vi "Galil Motion Controller (Keith Koch's conflicted copy 2013-05-10).vi"   [LabVIEW 2011]
uses:
  _GlobalVariables&Libraries/ATV Program Global Variables.vi
types:
  T1 = cluster{"Drive Value Output String":string, "Steer Value Output String":string, "Error Out":errorcluster, "Initial Encoder Counts":string, "Disable Galil Terminal":bool, "Command Input":string}
  T2 = cluster{"End ATV Program":bool, "E-Stop":bool, "Save Logfile":bool, "Logfile Iteration Delay (ms)":u32, "Loop iteration time (ms)":u32, "Logfile Location":path, "Default GPS Navigation Path":path, "Computer":string, "Default GPS Boundary Path":path}
  T3 = cluster{"Navigation Coordinates":cluster{"Latitude":dbl, "Longitude":dbl}[], "Coordinate Count":u32, "Drive Speed":string, "Steer Angle":dbl, "Steering":dbl, "Direction to next Coordinate":dbl, "Drive":dbl, "Navigation Path":string}
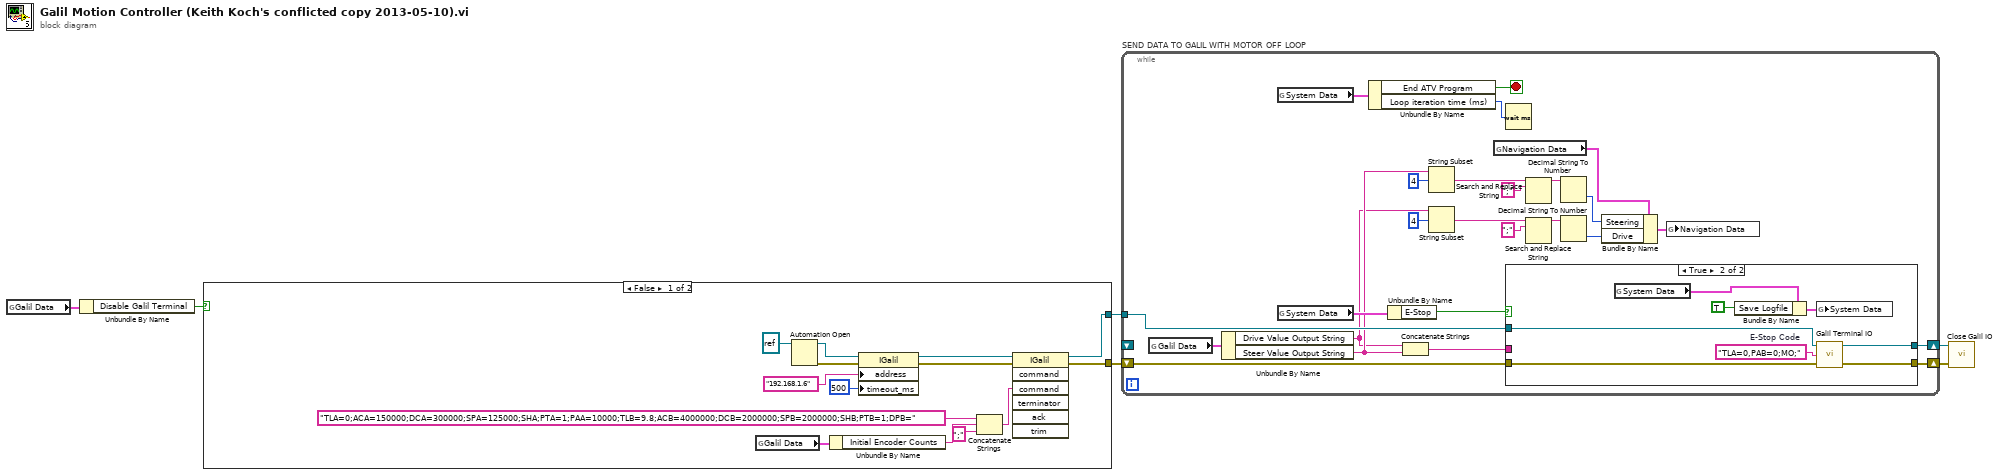
[diagram p0: block diagram]
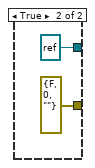
[diagram p2: hidden frame]
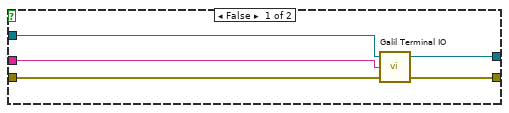
[diagram p3: hidden frame]
diagram:
  n1 = global read "ATV Program Global Variables.vi" "Galil Data"() -> (w4:T1)
  n2 = Unbundle By Name(w4) -> ("Disable Galil Terminal"=w3:bool)
  n3 = case shown="False" w3 {
    tunnel: [w14 refnum<k7> refnum ("Galil.IGalil")] -> w2
    tunnel: [w13 errorcluster {"status"=FALSE, "code"=0, "source"=""} ("error out")] -> w1
    frame False {
      n4 = global read "ATV Program Global Variables.vi" "Galil Data"() -> (w11:T1)
      n5 = Automation Open(Automation Refnum=refnum<k7> refnum ("Galil.IGalil")) -> (Automation Refnum=w19:refnum<k7>, error out=w18:errorcluster)  [unwired: 3 in]
      n6 = Unbundle By Name(w11) -> ("Initial Encoder Counts"=w10:string)
      n7 = property class="IGalil"(reference=w19, error in=w18, "address"="192.168.1.6", "timeout_ms"=500) -> (reference out=w8:refnum<k7>, error out=w7:errorcluster)
      n8 = Concatenate Strings("TLA=0;ACA=150000;DCA=300000;SPA=125000;SHA;PTA=1;PAA=10000;TLB=9.8;ACB=4000000;DCB=2000000;SPB=2000000;SHB;PTB=1;DPB=" ("Command Input"), w10, ";" ("string")) -> (w12:string)
      n9 = invoke class="IGalil" method="command"(reference=w8, error in=w7, "command"=w12) -> (reference out=w14:refnum<k7>, error out=w13:errorcluster)  [unwired: 4 in, 5 out]
    }
    frame True {
    }
  }
  n10 = while "SEND DATA TO GALIL WITH MOTOR OFF LOOP" {
    tunnel: w2 -> [w46]
    shift-right: [w43] -> w5
    shift-left: w1 -> [w44]
    shift-right: [w45] -> w6
    shift-left: _ -> [_]
    stop <- w38 stop-if-true
    n11 = global read "ATV Program Global Variables.vi" "Galil Data"() -> (w42:T1)
    n12 = Unbundle By Name(w42) -> ("Drive Value Output String"=w23:string, "Steer Value Output String"=w29:string)
    n13 = global read "ATV Program Global Variables.vi" "System Data"() -> (w39:T2)
    n14 = global read "ATV Program Global Variables.vi" "System Data"() -> (w41:T2)
    n15 = Unbundle By Name(w39) -> ("End ATV Program"=w38:bool, "Loop iteration time (ms)"=w37:u32)
    n16 = Unbundle By Name(w41) -> ("E-Stop"=w40:bool)
    n17 = Concatenate Strings(w23, w29) -> (w47:string)
    n18 = String Subset(string=w29, offset (0)=4) -> (substring=w34:string)  [unwired: 1 in]
    n19 = String Subset(string=w23, offset (0)=4) -> (substring=w27:string)  [unwired: 1 in]
    n20 = global read "ATV Program Global Variables.vi" "Navigation Data"() -> (w32:T3)
    n21 = Wait (ms)(milliseconds to wait=w37) -> ()  [unwired: 1 out]
    n22 = case shown="True" w40 {
      tunnel: w47 -> [w52 _]
      tunnel: w46 -> [w51 w58]
      tunnel: [w50 w60] -> w45
      tunnel: w44 -> [w49 w57]
      tunnel: [w48 w59] -> w43
      frame False {
        n23 = call "Galil Terminal IO.vi"("Galil Error In"=w49, "Command Input"=w52, "Reference In"=w51) -> ("Galil Error Out"=w48:errorcluster, "Reference Out"=w50:refnum<k7>)  [unwired: 1 out]
      }
      frame True {
        w56 = "TLA=0,PAB=0;MO;"  # E-Stop Code
        n24 = global read "ATV Program Global Variables.vi" "System Data"() -> (w54:T2)
        n25 = Bundle By Name(cluster=w54, "Save Logfile"=TRUE) -> (w55:T2)
        n26 = global write "ATV Program Global Variables.vi" "System Data"(w55) -> ()
        n27 = call "Galil Terminal IO.vi"("Galil Error In"=w57, "Command Input"=w56, "Reference In"=w58) -> ("Galil Error Out"=w59:errorcluster, "Reference Out"=w60:refnum<k7>)  [unwired: 1 out]
      }
    }
    n28 = Search and Replace String(input string=w34, search string=";") -> (result string=w35:string)  [unwired: 6 in, 3 out]
    n29 = Search and Replace String(input string=w27, search string=";") -> (result string=w26:string)  [unwired: 6 in, 3 out]
    n30 = Decimal String To Number(string=w35) -> (number=w31:i32)  [unwired: 2 in, 1 out]
    n31 = Decimal String To Number(string=w26) -> (number=w24:i32)  [unwired: 2 in, 1 out]
    n32 = Bundle By Name(cluster=w32, "Steering"=w31, "Drive"=w24) -> (w30:T3)
    n33 = global write "ATV Program Global Variables.vi" "Navigation Data"(w30) -> ()
  }
  n34 = call "Close Galil IO.vi"("Error In"=w5, "Reference In"=w6) -> ()  [unwired: 2 in, 2 out]
